vi "Obtain Task Notifiers and Queues.vi"(8 "error in (no error)":errorcluster, 11 "Task Base in":refnum<class "Task Base.lvclass">) -> (0 "error out":errorcluster, 3 "Task Base out":refnum<class "Task Base.lvclass">)   [LabVIEW 2023, in "HAL GOOP4.lvlib" / "Task Base.lvclass"]
uses:
  Task Base.lvclass
  Task Base.lvclass/Task Base.ctl
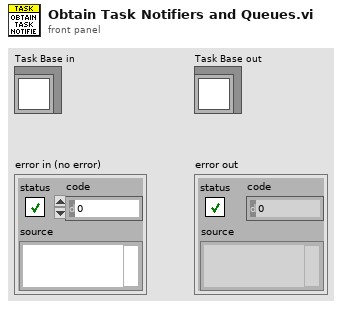
[diagram p1: front panel]
types:
  T1 = cluster{"Stop PE":refnum<notifier>, "Data":refnum<notifier>}
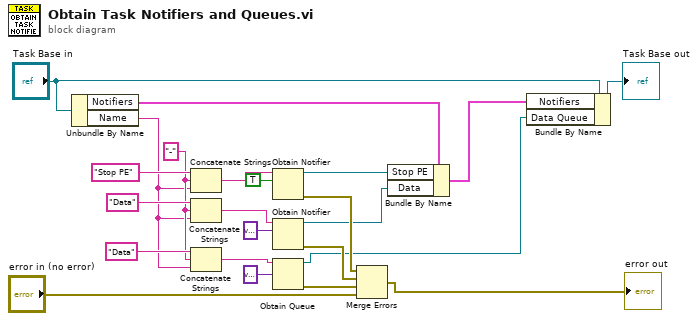
[diagram p0: block diagram]
diagram:
  w2 = "-" ("string")
  n1 = Unbundle By Name("Task Base in") -> ("Notifiers"=w9:T1, "Name"=w1:string)
  n2 = Concatenate Strings("Stop PE" ("name (unnamed)"), w2, w1) -> (w5:string)
  n3 = Concatenate Strings("Data" ("name (unnamed)"), w2, w1) -> (w4:string)
  n4 = Concatenate Strings("Data" ("name (unnamed)"), w2, w1) -> (w3:string)
  n5 = Obtain Notifier(name (unnamed)=w5, notification data type=TRUE) -> (notifier out=w12:refnum<notifier>, error out=w16:errorcluster)  [unwired: 2 in, 1 out]
  n6 = Obtain Notifier(name (unnamed)=w4, notification data type=variant) -> (notifier out=w11:refnum<notifier>, error out=w15:errorcluster)  [unwired: 2 in, 1 out]
  n7 = Obtain Queue(name (unnamed)=w3, element data type=variant) -> (queue out=w7:refnum<queue>, error out=w14:errorcluster)  [unwired: 3 in, 1 out]
  n8 = Merge Errors(w16, w15, w14, "error in (no error)") -> (→"error out":errorcluster)
  n9 = Bundle By Name(cluster=w9, "Stop PE"=w12, "Data"=w11) -> (w8:T1)
  n10 = Bundle By Name(cluster="Task Base in", "Notifiers"=w8, "Data Queue"=w7) -> (→"Task Base out":refnum<class "Task Base.lvclass">)
